vi "set move settings.vi"(8 "error in (no error)":errorcluster, 10 "move_settings":T1, 11 "id":i32) -> (0 "error out":errorcluster, 3 "function return":i32)   [LabVIEW 2012, in "libximc.lvlib"]
doc: "result_t XIMC_API set_move_settings (device_t id, const move_settings_t* move_settings);"
uses:
  libximc.lvlib
  libximc.dll
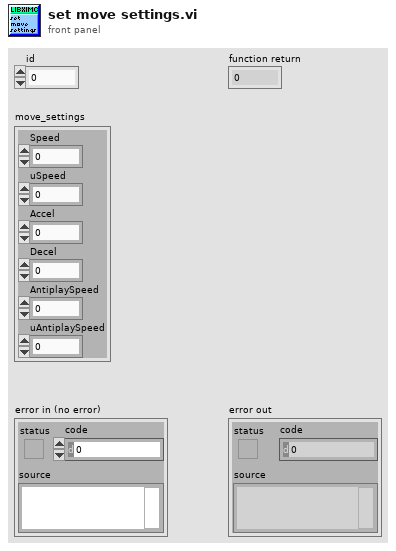
[diagram p1: front panel]
types:
  T1 = cluster{"Speed":u32, "uSpeed":u32, "Accel":u32, "Decel":u32, "AntiplaySpeed":u32, "uAntiplaySpeed":u32}
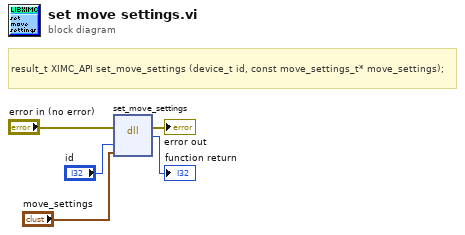
[diagram p0: block diagram]
diagram:
  # "result_t XIMC_API set_move_settings (device_t id, const move_settings_t* move_settings);"
  n1 = dll-call lib="C:/Users/user/Desktop/labview-2.9.11-gen/libximc.*" fn="set_move_settings"(error in="error in (no error)", "id"="id", "move_settings"="move_settings") -> (error out=→"error out":errorcluster, →"function return":i32)  [unwired: 4 in, 1 out]
